vi "TP1.1.vi"() -> ()   [LabVIEW 2013]
panel:
  out "Waveform Graph":dbl[](graph)
  in  "Cantidad de Muestras":i32=1000
  in  "Amplitud":dbl=10.0
  in  "Frecuencia":dbl=5.0
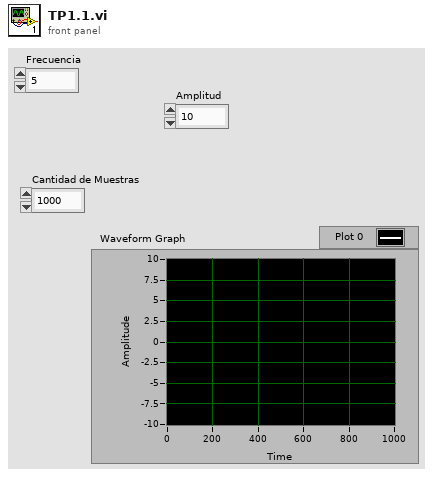
[diagram p1: front panel]
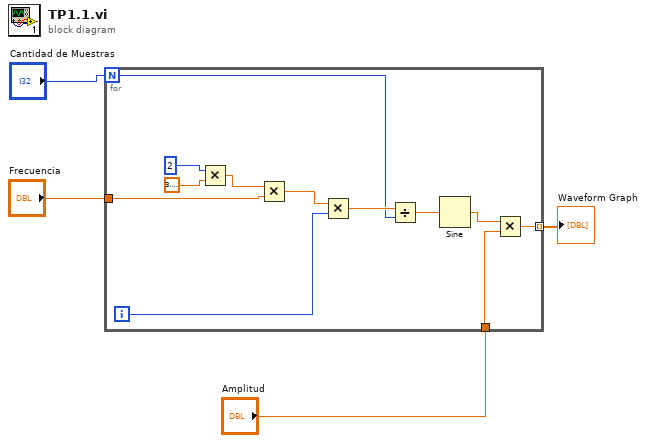
[diagram p0: block diagram]
diagram:
  n1 = for {
    N: "Cantidad de Muestras" -> [w11]
    tunnel: "Frecuencia" -> [w8]
    tunnel: "Amplitud" -> [w7]
    tunnel: [w5] -> w2 mode=indexing
    i -> [w9]
    n2 = Multiply(x=2, y=3.141592653589793) -> (x*y=w14:dbl)
    n3 = Multiply(x=w14, y=w8) -> (x*y=w13:dbl)
    n4 = Multiply(x=w13, y=w9) -> (x*y=w12:dbl)
    n5 = Divide(x=w12, y=w11) -> (x/y=w10:dbl)
    n6 = Sine(x=w10) -> (sin(x)=w6:dbl)
    n7 = Multiply(x=w6, y=w7) -> (x*y=w5:dbl)
  }
  "Waveform Graph" <- w2
